vi "Modbus_Scan_Test.vi"(8 "error in (no error)":errorcluster, 10 "channel":u8, 11 "MB_Master in":refnum<class "MB_Master.lvclass">) -> (0 "error out":errorcluster, 3 "MB_Master out":refnum<class "MB_Master.lvclass">)   [LabVIEW 2023, in "TranslationStage Library.lvlib" / "Jiaxin_Stepper_Controller.lvlib" / "Jiaxin_Stepper.lvclass"]
uses:
  Jiaxin_Stepper/Jiaxin_Stepper.lvclass
  <vilib>/Plasmionique/MB Master/MB_Master/MB_Master.lvclass
  <vilib>/Plasmionique/MB Master/MB Master.lvlib
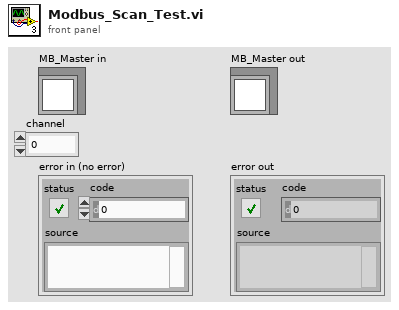
[diagram p1: front panel]
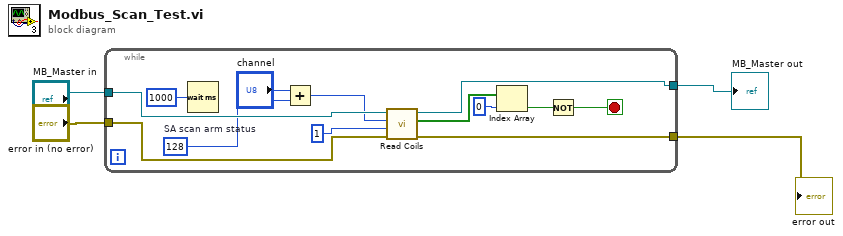
[diagram p0: block diagram]
diagram:
  n1 = while {
    tunnel: "error in (no error)" -> [w15]
    tunnel: [w14] -> w4
    tunnel: "MB_Master in" -> [w17]
    tunnel: [w16] -> w3
    stop <- w11 stop-if-true
    w7 = 128  # SA scan arm status
    n2 = Wait (ms)(milliseconds to wait=u32 1000) -> ()  [unwired: 1 out]
    n3 = Add(x="channel", y=w7) -> (x+y=w6:i32)
    n4 = call <vilib>:"Read Coils.vi"("error in (no error)"=w15, "quantity"=u16 1, "starting address"=w6, "MB session in"=w17) -> ("error out"=w14:errorcluster, "Coils"=w10:bool[], "MB session out"=w16:refnum<class "MB_Master.lvclass">)  [unwired: 5 in]
    n5 = Index Array(array=w10, index=0) -> (element=w8:bool)
    n6 = Not(x=w8) -> (.not. x?=w11:bool)
  }
  "error out" <- w4
  "MB_Master out" <- w3
